vi "ADS1256 Read.vi"(9 "pData":i32[](array[numeric])=array[4097 elements], 10 "Channel":i8, 11 "DevHandle":i32) -> (1 "pData out":i32[](array[numeric]), 3 "function return":i32)   [LabVIEW 2010, in "usb2ads1256.lvlib"]
doc: "int WINAPI ADS1256_Read(int DevHandle,char Channel,int *pData);"
uses:
  usb2ads1256.lvlib
  USB2XXX.dll
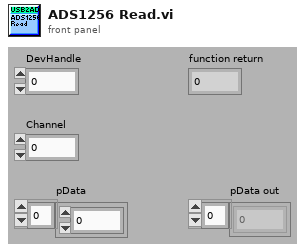
[diagram p1: front panel]
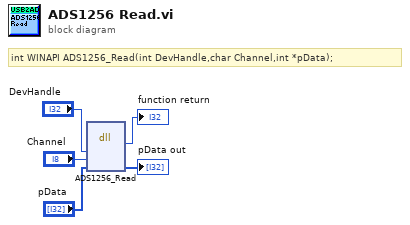
[diagram p0: block diagram]
diagram:
  # "int WINAPI ADS1256_Read(int DevHandle,char Channel,int *pData);"
  n1 = dll-call lib="G:/OtherWork/USB2XXX_Example/trunk/Labview/PublicFiles/USB2XXX.*" fn="ADS1256_Read"("DevHandle"="DevHandle", "Channel"="Channel", "pData"="pData") -> (→"function return":i32, "pData"=→"pData out":i32[])  [unwired: 5 in, 2 out]
